vi "Find Workspace.vi"(8 "Error In":errorcluster, 10 "Control In":T2={"I-O.lvclass"=refnum, "Motion.lvclass"=refnum, "Dispenser.lvclass"=refnum}, 11 "Carrier Tray in":refnum<class "8 inch Assembly Tray.lvclass">) -> (0 "Error Out":errorcluster, 1 "Workspace":T1, 2 "Control Out":T2, 3 "Carrier Tray Out":refnum<class "8 inch Assembly Tray.lvclass">)   [LabVIEW 2016, in "8 inch Assembly Tray.lvclass"]
uses:
  8 inch Assembly Tray.lvclass
  Controller/Controllers.ctl
  Controller/I-O/I-O.lvclass
  Controller/Motion/A3200/A3200.lvclass
  Controller/Dispenser/Dispenser.lvclass
  Controller/Motion/Motion.lvclass
  Workspace.ctl
  Carrier Tray/Assembly Tray.lvclass
  Controller/Controller.lvclass
  Fixture.lvclass
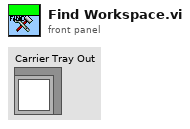
[diagram p1: front panel]
types:
  T1 = typedef "Fixture.lvclass/Workspace.ctl" = cluster{"XYZTheta":dbl[], "Workspace Valve":i32, "Workspace Sensor":i32}
  T2 = typedef "Controller.lvclass/Controllers.ctl" = cluster{"I-O.lvclass":refnum<class "I-O.lvclass">, "Motion.lvclass":refnum<class "Motion.lvclass">, "Dispenser.lvclass":refnum<class "Dispenser.lvclass">}
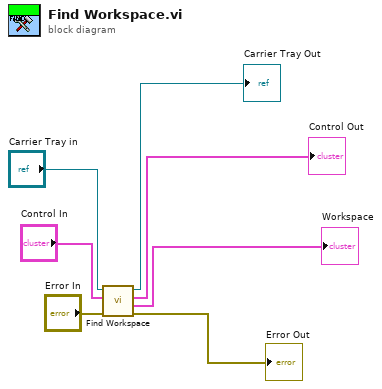
[diagram p0: block diagram]
diagram:
  n1 = call-parent "Find Workspace.vi"("Error In"="Error In", "Control In"="Control In", "Carrier Tray in"="Carrier Tray in") -> ("Error Out"=→"Error Out":errorcluster, "Workspace"=→"Workspace":T1, "Control Out"=→"Control Out":T2, "Carrier Tray Out"=→"Carrier Tray Out":refnum<class "8 inch Assembly Tray.lvclass">)  [unwired: 5 in]
